vi "LVPortGetPropertyUpdateParamNameAndTempID.vi"(10 "Event Data":variant, 11 "pID":string) -> (2 "Param Name":string, 3 "TempID":i32)   [LabVIEW 2017]
uses:
  Common/ObjectMap/LVPortObjectMapDataTypeEnum.ctl
  Common/ObjectMap/LVPortObjectMapContainerTypeEnum.ctl
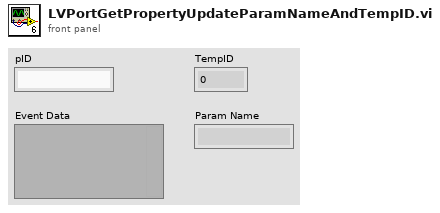
[diagram p1: front panel]
types:
  T1 = typedef "LVPortObjectMapContainerTypeEnum.ctl" = enum16{"Value", "Array", "Waveform"}
  T2 = typedef "LVPortObjectMapDataTypeEnum.ctl" = enum16{"NotAnObjectMapType", "Real", "Complex", "String", "Boolean"}
  T3 = typedef "LVPortObjectMapNamepathData.ctl" = cluster{"Type":T2, "Value":variant, "Namepath":string, "Typename":string, "Container Type":T1}
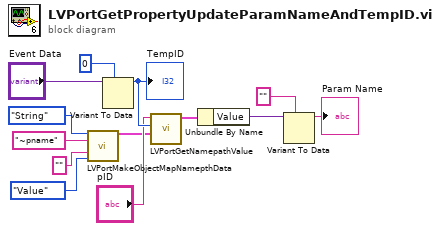
[diagram p0: block diagram]
diagram:
  n1 = call "LVPortMakeObjectMapNamepthData.vi"("ObjectMapType"=LVPortObjectMapDataTypeEnum."String" ("Type"), "namepath"="~pname" ("Namepath"), "value"="", "Labview Contriner type"=LVPortObjectMapContainerTypeEnum."Value") -> ("MatlabDataBundle"=w1:T3)  [unwired: 11 in]
  n2 = Variant To Data(type=0, Variant="Event Data") -> (data=w13:i32)  [unwired: 1 in, 1 out]
  "TempID" <- w13
  n3 = call "LVPortGetNamepathValue.vi"("Namepath Data in"=w1, "Object ID"=w13, "pID"="pID") -> ("Namepath Data out"=w9:T3)  [unwired: 6 in, 2 out]
  n4 = Unbundle By Name(w9) -> ("Value"=w11:variant)
  n5 = Variant To Data(type="", Variant=w11) -> (data=→"Param Name":string)  [unwired: 1 in, 1 out]
